vi "Filenamer.vi"(8 "error in":errorcluster, 9 "Method Version Folder":path, 10 "Design exists":bool, 11 "request variables":T1) -> (0 "error out":errorcluster, 3 "Project Folder":path)   [LabVIEW 2011, in "Design Server.lvlib"]
uses:
  AguaClara Design Server/Design Server.lvlib
  ADT 2/user project design.ctl
  AguaClara Design Server/Folders.ctl
panel:
  out "current time":timestamp
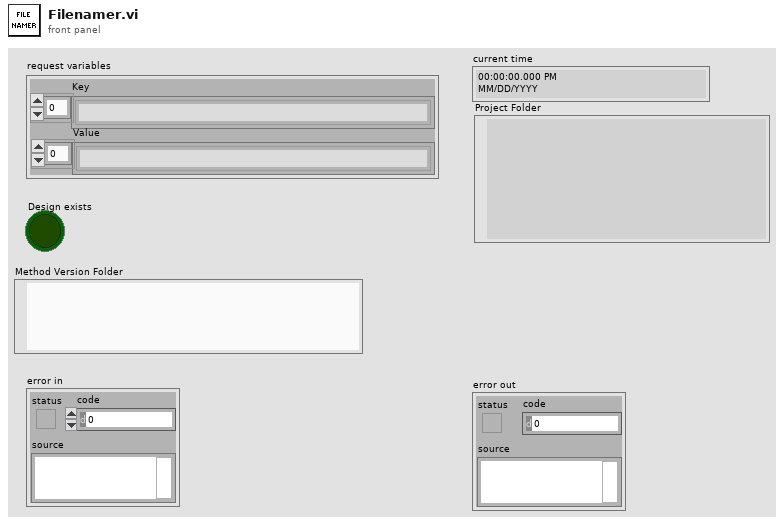
[diagram p1: front panel]
types:
  T1 = typedef "user project design.ctl" = cluster{"Key":string[], "Value":string[]}
  T2 = typedef "Design Server.lvlib/Folders.ctl" = enum16{"MathcadMethods", "RequestedDesigns", "CompletedDesigns", "MathcadCode", "CollabnetSVN.exe"}
  T3 = enum16{"open", "replace", "create", "open or create", "replace or create", "replace or create with confirmation"}
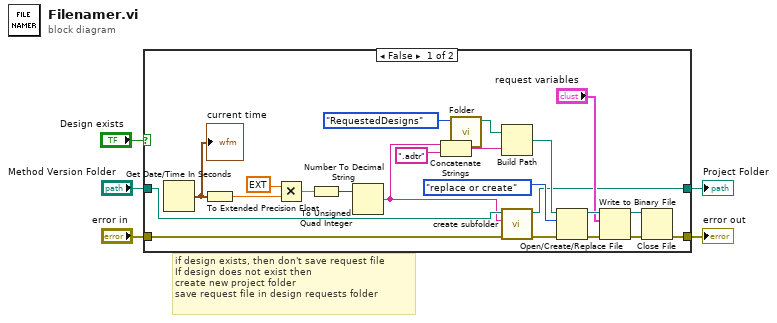
[diagram p0: block diagram]
diagram:
  # "if design exists, then don't save request file\nIf design does not exist then \ncreate new project folder\nsave request file in design requests folder"
  n1 = case shown="False" "Design exists" {
    tunnel: [w8 w29] -> w5
    tunnel: [w15 w28] -> w4
    tunnel: "Method Version Folder" -> [w10 w29]
    tunnel: "error in" -> [w7 w28]
    frame False {
      n2 = Get Date/Time In Seconds() -> (seconds since 1Jan1904=w27:timestamp)
      "current time" <- w27
      n3 = To Extended Precision Float(1:w27) -> (0:w26:ext)
      n4 = Multiply(x=ext 100.0, y=w26) -> (x*y=w24:ext)
      n5 = To Unsigned Quad Integer(1:w24) -> (0:w23:u64)
      n6 = Number To Decimal String(number=w23) -> (decimal integer string=w9:string)  [unwired: 1 in]
      n7 = Concatenate Strings(w9, ".adtr" ("string")) -> (w12:string)
      n8 = call "Folder.vi"("Folders"=Folders."RequestedDesigns") -> ("FolderPath"=w13:path)  [unwired: 8 in, 2 out]
      n9 = Build Path(base path=w13, name or relative path=w12) -> (appended path=w11:path)
      n10 = call "create subfolder.vi"("error in (no error)"=w7, "Folder Name"=w9, "FolderPath"=w10) -> ("error out"=w6:errorcluster, "Subfolder path"=w8:path)  [unwired: 7 in]
      n11 = Open/Create/Replace File(file path (use dialog)=w11, error in=w6, operation (0:open)=T3."replace or create") -> (refnum out=w18:refnum<file>, error out=w16:errorcluster)  [unwired: 3 in, 1 out]
      n12 = Write to Binary File(file (use dialog)=w18, data="request variables", error in=w16) -> (refnum out=w20:refnum<file>, error out=w19:errorcluster)  [unwired: 3 in, 1 out]
      n13 = Close File(refnum=w20, error in=w19) -> (error out=w15:errorcluster)  [unwired: 1 out]
    }
    frame True {
    }
  }
  "error out" <- w4
  "Project Folder" <- w5
